vi "Untitled 2.vi"() -> ()   [LabVIEW 2018]
panel:
  in  "muilt":dbl=1.0
  out "x*y":dbl[](array[numeric])=[-0.5000000000000001, -0.4500000000000001, -0.10000000000000002, 0.0]
  in  "Array":dbl[](array[numeric])=[-1.0, -0.9, -0.2, 0.0]
  out "exp(x)":dbl[](array[numeric])=[0.6065306597126333, 0.6376281516217732, 0.9048374180359595, 1.0]
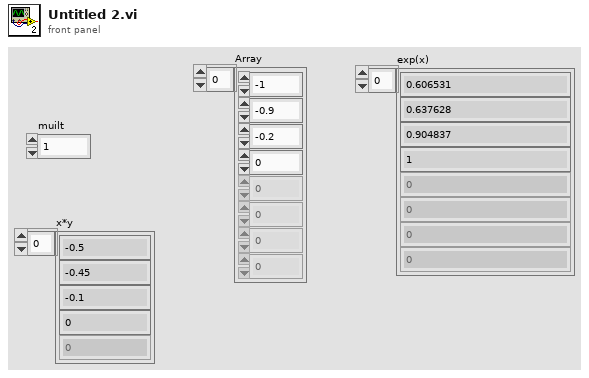
[diagram p1: front panel]
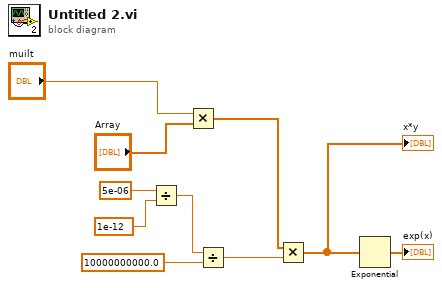
[diagram p0: block diagram]
diagram:
  n1 = Divide(x=5e-06, y=1e-12) -> (x/y=w8:dbl)
  n2 = Multiply(x="muilt", y="Array") -> (x*y=w1:dbl[])
  n3 = Divide(x=w8, y=10000000000.0) -> (x/y=w6:dbl)
  n4 = Multiply(x=w1, y=w6) -> (x*y=w5:dbl[])
  "x*y" <- w5
  n5 = Exponential(1:w5) -> (0:→"exp(x)":dbl[])
